vi "Increment Indexes.vi"(5 "group index to increment":i32, 7 "lengths":u8[](array[numeric]), 10 "max indexes":u8[](array[numeric]), 11 "previous indexes":u8[](array[numeric])) -> (2 "complete":bool, 3 "next indexes":u8[](array[numeric]))   [LabVIEW 2022 SP3]
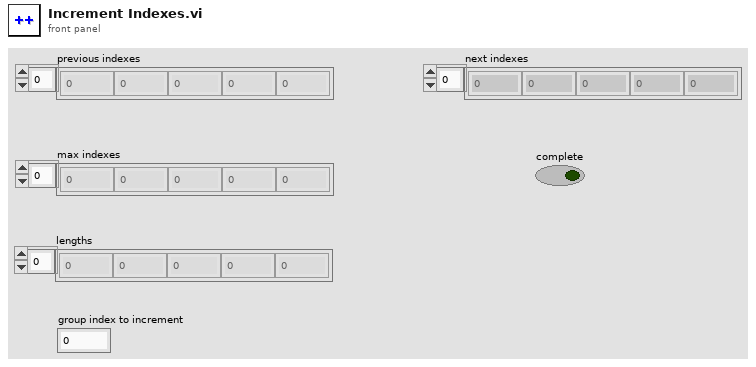
[diagram p1: front panel]
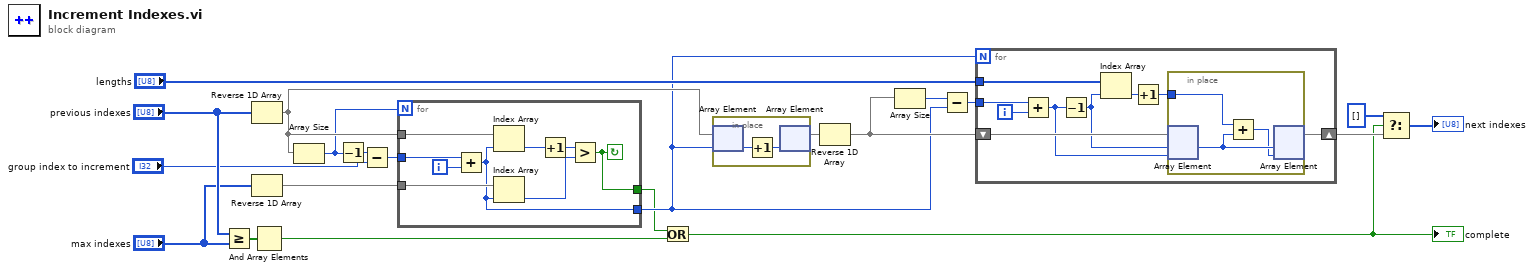
[diagram p0: block diagram]
diagram:
  n1 = Greater Or Equal?(x="previous indexes", y="max indexes") -> (x >= y?=w21:bool[])
  n2 = Reverse 1D Array(array="previous indexes") -> (reversed array=w13:u8[])
  n3 = Reverse 1D Array(array="max indexes") -> (reversed array=w15:u8[])
  n4 = And Array Elements(Boolean array=w21) -> (logical AND=w6:bool)
  n5 = Array Size(array=w13) -> (size(s)=w5:i32)
  n6 = Decrement(x=w5) -> (x-1=w12:i32)
  n7 = Subtract(x=w12, y="group index to increment") -> (x-y=w8:i32)
  n8 = for {
    N: w5 -> [_]
    tunnel: w13 -> [w28]
    tunnel: w15 -> [w26]
    tunnel: [w23] -> w10
    tunnel: w8 -> [w24]
    tunnel: [w22] -> w7
    i -> [w25]
    stop <- w22 continue-if-true
    n9 = Add(x=w24, y=w25) -> (x+y=w23:i32)
    n10 = Index Array(array=w28, index=w23) -> (element=w29:u8)
    n11 = Index Array(array=w26, index=w23) -> (element=w27:u8)
    n12 = Increment(x=w29) -> (x+1=w30:u8)
    n13 = Greater?(x=w30, y=w27) -> (0:w22:bool)
  }
  n14 = Or(x=w7, y=w6) -> (x .or. y?=w3:bool)
  "complete" <- w3
  n15 = in-place {
    n16 = in-place-array #1(w13, w10) -> (w32:u8)
    n17 = Increment(x=w32) -> (x+1=w31:u8)
    n18 = in-place-array #1(w31) -> (w14:u8[])  [unwired: 1 out]
  }
  n19 = Reverse 1D Array(array=w14) -> (reversed array=w16:u8[])
  n20 = Array Size(array=w16) -> (size(s)=w17:i32)
  n21 = Subtract(x=w17, y=w10) -> (x-y=w9:i32)
  n22 = for {
    N: w10 -> [_]
    shift-right: [w33] -> w4
    shift-left: w16 -> [w41]
    tunnel: w9 -> [w39]
    tunnel: "lengths" -> [w36]
    i -> [w40]
    n23 = Add(x=w39, y=w40) -> (x+y=w38:i32)
    n24 = Decrement(x=w38) -> (x-1=w37:i32)
    n25 = Index Array(array=w36, index=w37) -> (element=w35:u8)
    n26 = Increment(x=w35) -> (x+1=w34:u8)
    n27 = in-place {
      in-place-border: w34 -> [w43]
      n28 = in-place-array #2(w41, w37, w38) -> (w44:u8)  [unwired: 1 out]
      n29 = Add(x=w43, y=w44) -> (x+y=w42:u8)
      n30 = in-place-array #2(w44, w42) -> (w33:u8[])  [unwired: 2 out]
    }
  }
  n31 = Select(t=u8[] [], s=w3, f=w4) -> (s? t:f=→"next indexes":u8[])
